vi "Read Plot Array.vi"(8 "error in (no error)":errorcluster, 11 "2D Plot in":refnum<class "2D Plot.lvclass">) -> (0 "error out":errorcluster, 1 "Plot Property Array":T1, 3 "2D Plot out":refnum<class "2D Plot.lvclass">)   [LabVIEW 2020, in "2D Plot.lvclass"]
uses:
  <vilib>/Math Plots/2D Math Plots/2D Plot/2D Plot/2D Plot.lvclass
  <vilib>/Math Plots/2D Math Plots/2D Plot/2D Plot/Typedef/Plot Property Array.ctl
  <vilib>/Math Plots/2D Math Plots/2D Plot/2D Plot/Typedef/Plot Property.ctl
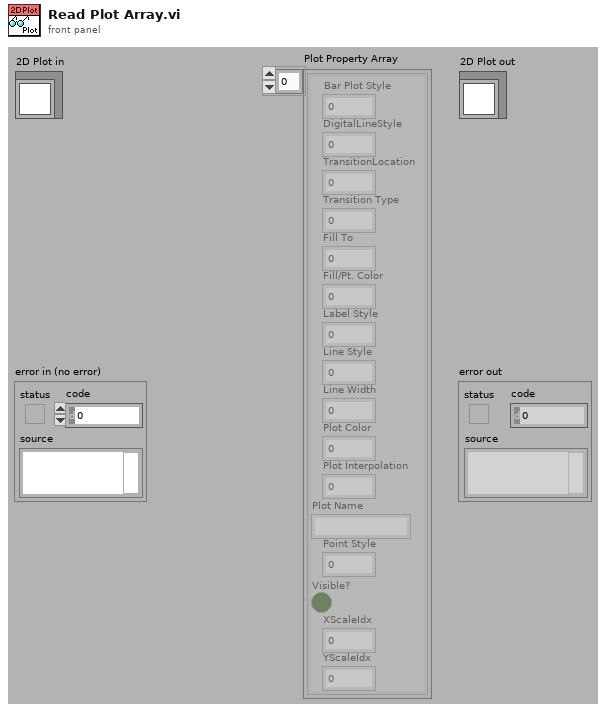
[diagram p1: front panel]
types:
  T1 = typedef "2D Plot.lvclass/Plot Property Array.ctl" = T2[]
  T2 = typedef "2D Plot.lvclass/Plot Property.ctl" = cluster{"Bar Plot Style":u8, "DigitalLineStyle":u8, "TransitionLocation":u8, "Transition Type":u8, "Fill To":i16, "Fill/Pt. Color":u32, "Label Style":u8, "Line Style":u8, "Line Width":u8, "Plot Color":u32, "Plot Interpolation":u8, "Plot Name":string, "Point Style":u8, "Visible?":bool, "XScaleIdx":u32, "YScaleIdx":u32}
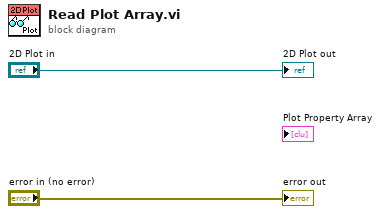
[diagram p0: block diagram]
diagram:
  "error out" <- "error in (no error)"
  "2D Plot out" <- "2D Plot in"
